vi "Save_to_Project.vi"(8 "error in (no error)":errorcluster, 9 "index":i32, 10 "buildObject":T1, 11 "AB_Source_Library in":refnum<class "AB_Source_Library.lvclass">) -> (0 "error out":errorcluster, 3 "AB_Source_Library out":refnum<class "AB_Source_Library.lvclass">)   [LabVIEW 2020, in "AB_Source_Library.lvclass"]
uses:
  <vilib>/AppBuilder/AB_Classes/Source/Library/AB_Source_Library.lvclass
  <resource>/Framework/Providers/API/ItemRef.ctl
  <vilib>/AppBuilder/RW_Project/AB_RW_Project_Source_Library_Data.ctl
  <vilib>/AppBuilder/RW_Project/AB_RW_Project_PropBag_Action.ctl
  <vilib>/AppBuilder/AB_Classes/Source/Library/AB_Source_Library.lvclass/AB_Source_Library.ctl
  <vilib>/AppBuilder/AB_Classes/Source/AB_Source.lvclass
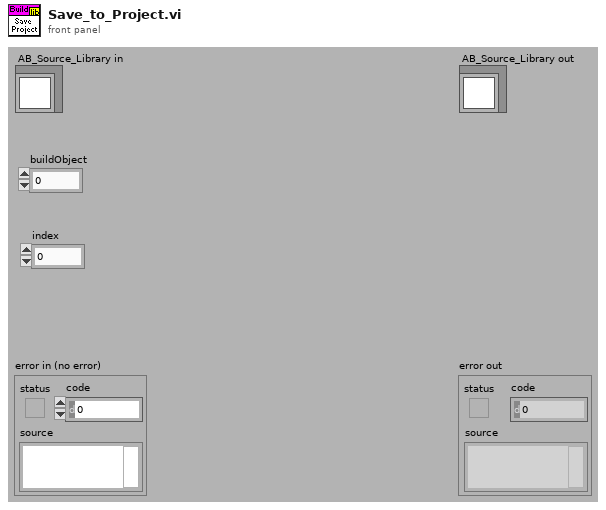
[diagram p1: front panel]
types:
  T1 = typedef "ItemRef.ctl" = u64
  T2 = typedef "AB_RW_Project_Source_Library_Data.ctl" = cluster{"relinkCallers":bool, "atomicCopy":bool, "allowMissingMembers":bool, "LVLIBPtopLevel":bool}
  T3 = typedef "AB_RW_Project_PropBag_Action.ctl" = enum16{"read", "write", "clear", "readPrevious", "writePrevious", "clearPrevious"}
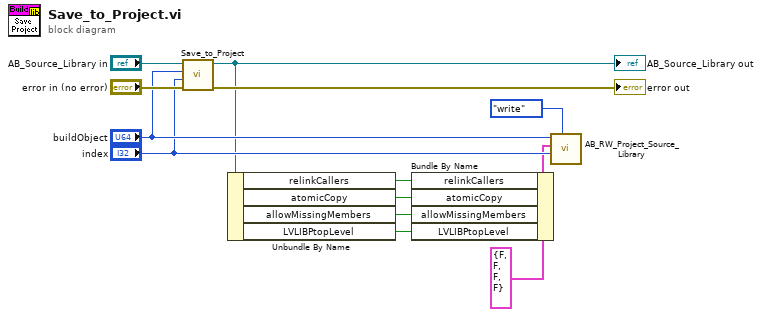
[diagram p0: block diagram]
diagram:
  n1 = call-parent "Save_to_Project.vi"("error in (no error)"="error in (no error)", "index"="index", "buildObject"="buildObject", "AB_Source in"="AB_Source_Library in") -> ("error out"=→"error out":errorcluster, "AB_Source out"=w6:refnum<class "AB_Source_Library.lvclass">)  [unwired: 6 in]
  "AB_Source_Library out" <- w6
  n2 = Unbundle By Name(w6) -> ("relinkCallers"=w5:bool, "atomicCopy"=w4:bool, "allowMissingMembers"=w2:bool, "LVLIBPtopLevel"=w1:bool)
  n3 = Bundle By Name(cluster=T2 {"relinkCallers"=FALSE, "atomicCopy"=FALSE, "allowMissingMembers"=FALSE, "LVLIBPtopLevel"=FALSE} ("dataSource in"), "relinkCallers"=w5, "atomicCopy"=w4, "allowMissingMembers"=w2, "LVLIBPtopLevel"=w1) -> (w3:T2)
  n4 = call <vilib>:"AB_RW_Project_Source_Library.vi"("action"=AB_RW_Project_PropBag_Action."write", "index in"="index", "dataSource in"=w3, "buildObject"="buildObject") -> ()  [unwired: 4 in, 4 out]
